vi "RotateToPosX.vi"(1 "P":cluster{"x":dbl, "y":dbl, "z":dbl}={"x"=-4.0, "y"=0.0, "z"=4.0} {"x" format="%.2f"; "z" format="%.2f"; "y" format="%.2f"}) -> (0 "Rotatation Matrix":dbl[][](array[numeric]) format="%.2f")   [LabVIEW 2022 SP3]
uses:
  <vilib>/Analysis/baseanly.llb/A x Vector.vi
  <vilib>/Analysis/NI_AALPro.lvlib
  <vilib>/Analysis/NI_AALBase.lvlib
panel:
  out "A x Vector":dbl[](array[numeric]) format="%.2f"
  # "Find rotation matrix to move vector P to point in the +x direction. The columns in rotation matrix indicate where new x'y'z' axis point. When rotated they point in xyz direction."
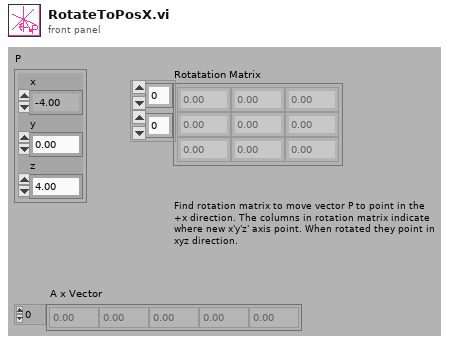
[diagram p1: front panel]
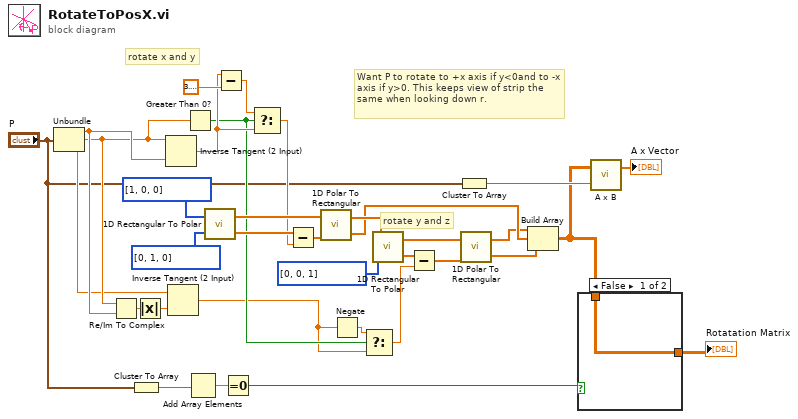
[diagram p0: block diagram]
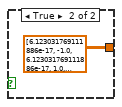
[diagram p2: hidden frame]
diagram:
  # "Want P to rotate to +x axis if y<0and to -x axis if y>0. This keeps view of strip the same when looking down r."
  # "rotate y and z"
  # "rotate x and y"
  n1 = Unbundle("P") -> ("x"=w19:dbl, "y"=w18:dbl, "z"=w11:dbl)
  n2 = Re/Im To Complex(1:w19, 2:w18) -> (0:w24:cdb)
  n3 = Cluster To Array(cluster="P") -> (array=w5:dbl[])
  n4 = Absolute Value(x=w24) -> (abs(x)=w20:dbl)
  n5 = Inverse Tangent (2 Input)(1:w19, 2:w18) -> (0:w12:dbl)
  n6 = Inverse Tangent (2 Input)(1:w20, 2:w11) -> (0:w8:dbl)
  n7 = Greater Than 0?(x=w18) -> (x > 0?=w9:bool)
  n8 = Add Array Elements(numeric array=w5) -> (sum=w4:dbl)
  n9 = call <vilib>:"1D Rectangular To Polar.vi"("X"=i32[] [1, 0, 0] ("A x Vector 2"), "Y"=i32[] [0, 1, 0] ("A x Vector 2")) -> ("Magnitude"=w32:dbl[], "Phase"=w34:dbl[])  [unwired: 1 out]
  n10 = Subtract(x=w12, y=3.141592653589793) -> (x-y=w16:dbl)
  n11 = Equal To 0?(x=w4) -> (x = 0?=w3:bool)
  n12 = Select(t=w16, s=w9, f=w12) -> (s? t:f=w17:dbl)
  n13 = Subtract(x=w34, y=w17) -> (x-y=w33:dbl[])
  n14 = call <vilib>:"1D Polar To Rectangular.vi"("Magnitude"=w32, "Phase"=w33) -> ("X"=w23:dbl[], "Y"=w22:dbl[])  [unwired: 1 out]
  n15 = Negate(x=w8) -> (-x=w7:dbl)
  n16 = Select(t=w7, s=w9, f=w8) -> (s? t:f=w10:dbl)
  n17 = call <vilib>:"1D Rectangular To Polar.vi"("X"=w23, "Y"=i32[] [0, 0, 1] ("A x Vector 2")) -> ("Magnitude"=w29:dbl[], "Phase"=w31:dbl[])  [unwired: 1 out]
  n18 = Subtract(x=w31, y=w10) -> (x-y=w30:dbl[])
  n19 = Cluster To Array(cluster="P") -> (array=w15:dbl[])
  n20 = call <vilib>:"1D Polar To Rectangular.vi"("Magnitude"=w29, "Phase"=w30) -> ("X"=w21:dbl[], "Y"=w28:dbl[])  [unwired: 1 out]
  n21 = Build Array(w21, w22, w28) -> (w1:dbl[][])
  n22 = case shown="False" w3 {
    tunnel: [w35 dbl[][] [[6.123031769111886e-17, -1.0, 6.123031769111886e-17], [1.0, 1.2246063538223773e-16, 0.0], [0.0, 1.2246063538223773e-16, 1.0]] ("Rotatation Matrix")] -> w2
    tunnel: w1 -> [w35 _]
    frame False {
    }
    frame True {
    }
  }
  "Rotatation Matrix" <- w2
  n23 = call-poly <vilib>:"A x B.vi"("Vector"=w15, "A"=w1) -> ("A x Vector"=→"A x Vector":dbl[])  [unwired: 1 out]
